vi "Semaforo.vi"() -> ()   [LabVIEW 2016]
panel:
  in  "Stop Button 2":bool
  out "number (0 to 1) 2":dbl(graph)
  out "number (0 to 1)":dbl(graph)
  in  "Stop Button":bool
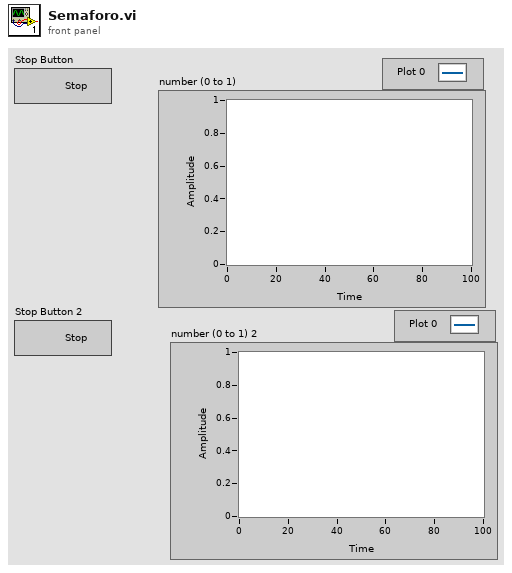
[diagram p1: front panel]
types:
  T1 = typedef "Semaphore RefNum" = refnum<k1>
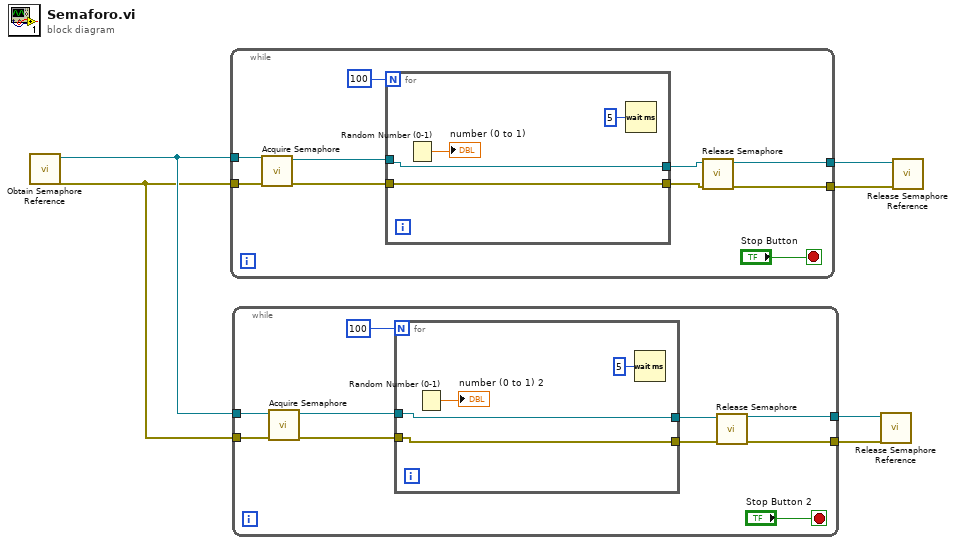
[diagram p0: block diagram]
diagram:
  n1 = call <vilib>:"Obtain Semaphore Reference.vi"() -> ("error out"=w5:errorcluster, "semaphore"=w6:T1)  [unwired: 5 in, 1 out]
  n2 = while {
    tunnel: w6 -> [w14]
    tunnel: w5 -> [w13]
    tunnel: [w8] -> w4
    tunnel: [w7] -> w3
    stop <- "Stop Button" stop-if-true
    n3 = call <vilib>:"Acquire Semaphore.vi"("error in (no error)"=w13, "semaphore"=w14) -> ("error out"=w11:errorcluster, "semaphore out"=w12:T1)  [unwired: 3 in, 1 out]
    n4 = for {
      N: u32 100 ("milliseconds to wait") -> [_]
      tunnel: w12 -> [w17]
      tunnel: w11 -> [w18]
      tunnel: [w18] -> w10
      tunnel: [w17] -> w9
      n5 = Random Number (0-1)() -> (number: 0 to 1=→"number (0 to 1)":dbl)
      n6 = Wait (ms)(milliseconds to wait=u32 5) -> ()  [unwired: 1 out]
    }
    n7 = call <vilib>:"Release Semaphore.vi"("error in (no error)"=w10, "semaphore"=w9) -> ("error out"=w7:errorcluster, "semaphore out"=w8:T1)  [unwired: 4 in]
  }
  n8 = while {
    tunnel: w6 -> [w28]
    tunnel: w5 -> [w27]
    tunnel: [w22] -> w2
    tunnel: [w21] -> w1
    stop <- "Stop Button 2" stop-if-true
    n9 = call <vilib>:"Acquire Semaphore.vi"("error in (no error)"=w27, "semaphore"=w28) -> ("error out"=w25:errorcluster, "semaphore out"=w26:T1)  [unwired: 3 in, 1 out]
    n10 = for {
      N: u32 100 ("milliseconds to wait") -> [_]
      tunnel: w26 -> [w32]
      tunnel: w25 -> [w31]
      tunnel: [w32] -> w24
      tunnel: [w31] -> w23
      n11 = Random Number (0-1)() -> (number: 0 to 1=→"number (0 to 1) 2":dbl)
      n12 = Wait (ms)(milliseconds to wait=u32 5) -> ()  [unwired: 1 out]
    }
    n13 = call <vilib>:"Release Semaphore.vi"("error in (no error)"=w23, "semaphore"=w24) -> ("error out"=w21:errorcluster, "semaphore out"=w22:T1)  [unwired: 4 in]
  }
  n14 = call <vilib>:"Release Semaphore Reference.vi"("error in (no error)"=w1, "semaphore"=w2) -> ()  [unwired: 8 in, 2 out]
  n15 = call <vilib>:"Release Semaphore Reference.vi"("error in (no error)"=w3, "semaphore"=w4) -> ()  [unwired: 8 in, 2 out]
